vi "ODE-PredatorPreyRHS.vi"(2 "data":variant, 3 "t":dbl, 4 "x1, x2,...":dbl[](array[numeric])) -> (0 "error out":errorcluster, 1 "f'(x)":dbl[](array[numeric]))   [LabVIEW 2023]
doc: "This VI contains the formula of the Predator-Prey ODE system model to be called by reference by the polymorphic ODE solver in VI mode. The Predator-Prey system can be described by the following equations:\n\ndx1/dt = ax1 - bx1x2\ndx2/dt = -cx2 + dx1x2\n\nIn this formula, x1(t) is the population of the prey and x2(t) is the population of the predators at a given point in time."
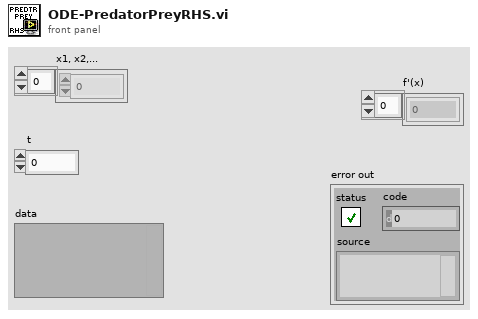
[diagram p1: front panel]
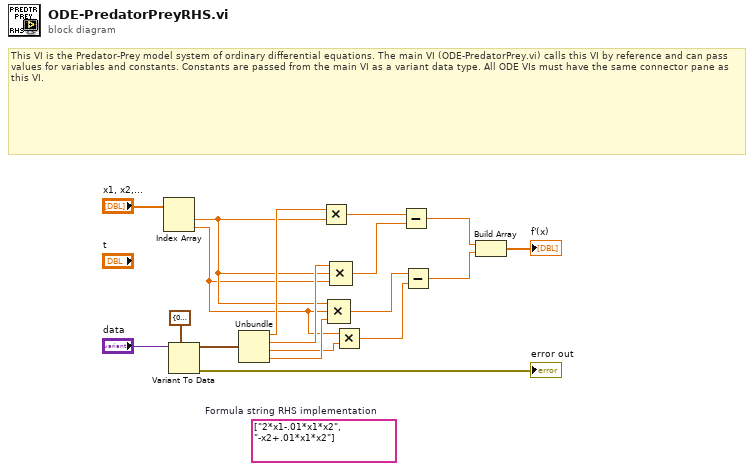
[diagram p0: block diagram]
diagram:
  (unwired) string[] ["2*x1-.01*x1*x2", "-x2+.01*x1*x2"]  # Formula string RHS implementation
  # "This VI is the Predator-Prey model system of ordinary differential equations. The main VI (ODE-PredatorPrey.vi) calls this VI by reference and can pass values for variables and constants. Constants are passed from the main VI as a variant data type. All ODE VIs must have the same connector pane as this VI."
  n1 = Index Array(array="x1, x2,...") -> (element #1=w8:dbl, element #2=w4:dbl)  [unwired: 2 in]
  n2 = Variant To Data(type=cluster{"x":dbl, "x":dbl, "x":dbl, "x":dbl} {"x"=0.0, "x"=0.0, "x"=0.0, "x"=0.0} ("output cluster"), Variant="data") -> (data=w11:cluster{"x":dbl, "x":dbl, "x":dbl, "x":dbl}, error out=→"error out":errorcluster)  [unwired: 1 in]
  n3 = Unbundle(w11) -> ("x"=w10:dbl, "x"=w9:dbl, "x"=w5:dbl, "x"=w7:dbl)
  n4 = Multiply(x=w10, y=w8) -> (x*y=w17:dbl)
  n5 = Compound Arithmetic op=MULTIPLY(w8, w4, w7) -> (w6:dbl)
  n6 = Compound Arithmetic op=MULTIPLY(w9, w8, w4) -> (w16:dbl)
  n7 = Multiply(x=w4, y=w5) -> (x*y=w3:dbl)
  n8 = Subtract(x=w17, y=w16) -> (x-y=w15:dbl)
  n9 = Subtract(x=w6, y=w3) -> (x-y=w14:dbl)
  n10 = Build Array(w15, w14) -> (→"f'(x)":dbl[])
